vi "SensorInterface_Main.vi"(8 "error in (no error)":errorcluster) -> (0 "error out":errorcluster)   [LabVIEW 2013]
doc: "This is Top Level VI for Sensor Interface Module. You can communicate with this module using its API. Communication is made based on queue. This module has User Interface so I chase Producer Consumer architecture. In this architecture the User Interface loop is closed using User Event. User Event is sent by Processing (Consumer) loop."
uses:
  General/Controls/#TD_General_CommunicationQueueStates_Enum.ctl
  Private controls/#TD_SensorInterface_InnerData_Cluster.ctl
  Private controls/#TD_SensorInterface_ModuleStates_Enum.ctl
  Private controls/#TD_SensorInterface_ModuleData_Cluster.ctl
  General/Controls/#TD_General_FromWho_Enum.ctl
  General/Controls/#TD_General_UserEventStates_Enum.ctl
panel:
  in  "Funds Dispensed":bool
  in  "DepositReceived":bool
  # "[Covers: UI4] \n[Covers: UI4A] \n[Covers: UI4B]"
  # "[Covers: UI1]"
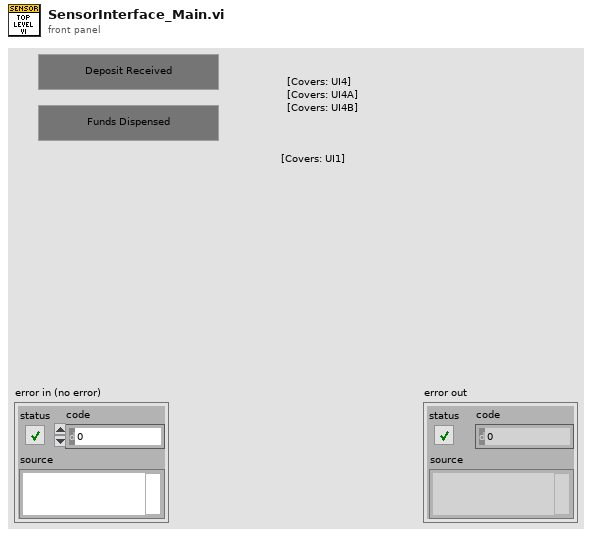
[diagram p1: front panel]
types:
  T1 = typedef "#TD_General_UserEventStates_Enum.ctl" = enum16{"ERROR_Default", "Create", "GetRef", "Generate", "Release"}
  T2 = typedef "#TD_General_CommunicationQueueStates_Enum.ctl" = enum16{"ERROR_Default", "Obtain", "GetRef", "Enqueue", "EnqueueAtOpp", "GetStatus", "Release"}
  T3 = typedef "#TD_General_FromWho_Enum.ctl" = enum16{"ERROR_Default", "UserConsole", "DisplayConsole", "SensorInterface", "Controller", "Database", "Timing", "ErrorHandling"}
  T4 = typedef "#TD_SensorInterface_ModuleStates_Enum.ctl" = enum16{"ERROR_Default", "Init", "Close", "ErrorHandling", "DepositReceived", "FundsDispensed"}
  T5 = typedef "#TD_SensorInterface_ModuleData_Cluster.ctl" = cluster{"Action":T4, "Data":variant}
  T6 = typedef "#TD_General_IntermoduleData_Cluster.ctl" = cluster{"Sender":T3, "ModuleData":variant}
  T7 = typedef "#TD_SensorInterface_InnerData_Cluster.ctl" = cluster{"Sth":bool}
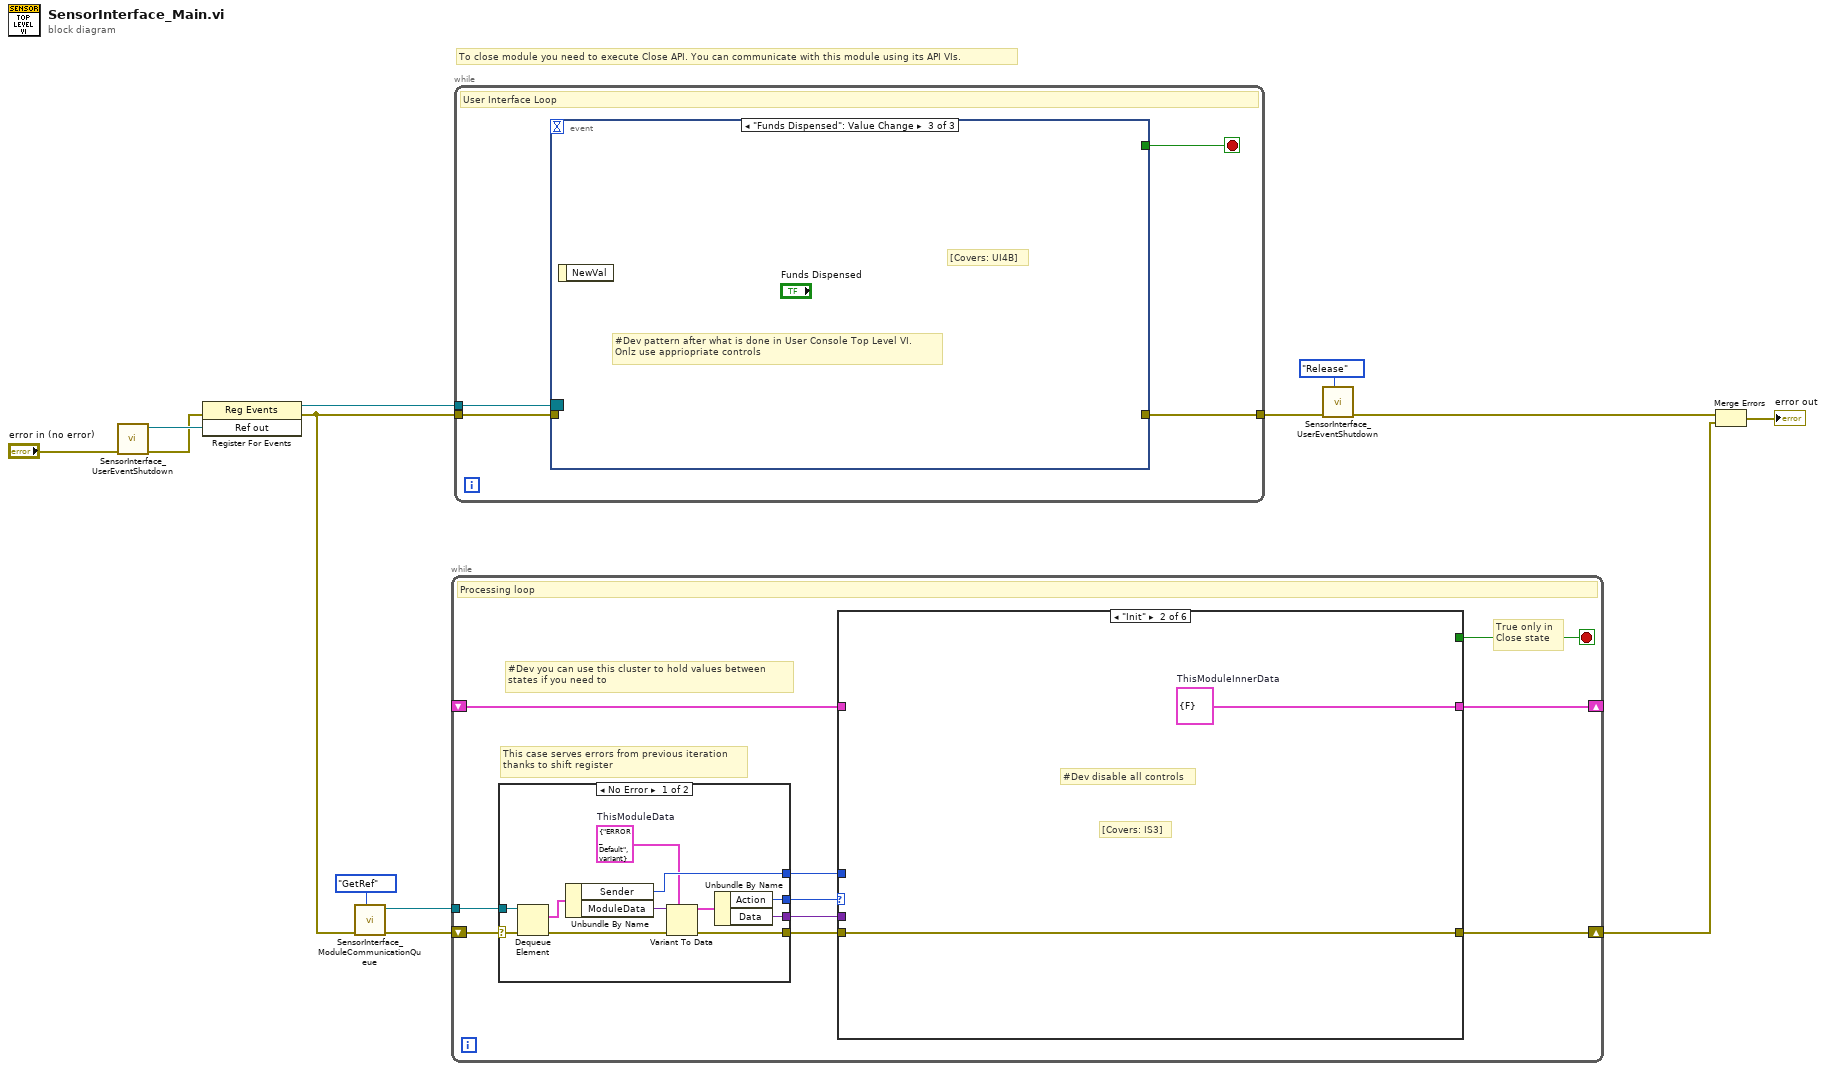
[diagram p0: block diagram]
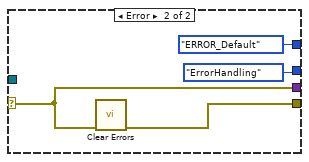
[diagram p2: hidden frame]
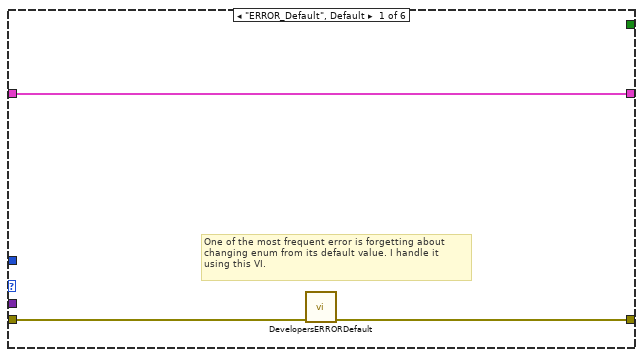
[diagram p3: hidden frame]
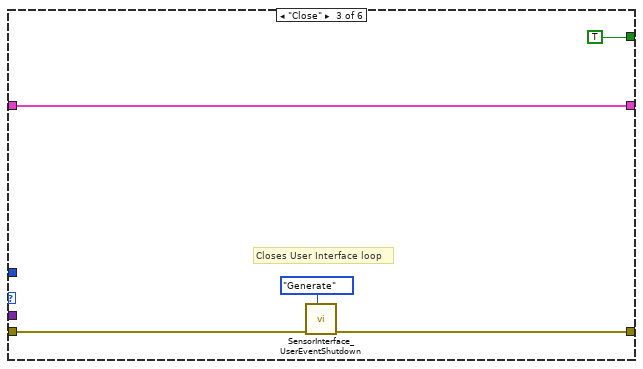
[diagram p4: hidden frame]
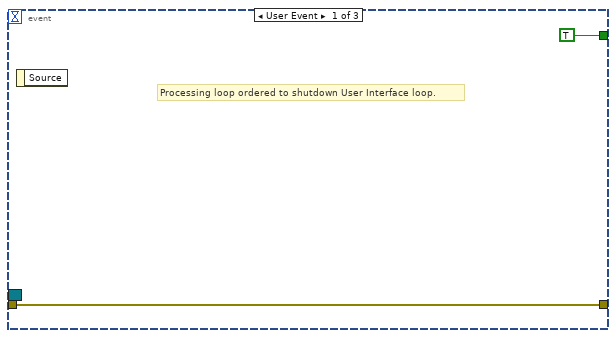
[diagram p8: hidden frame]
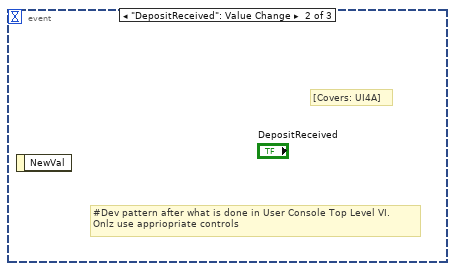
[diagram p9: hidden frame]
diagram:
  # "To close module you need to execute Close API. You can communicate with this module using its API VIs."
  n1 = call "SensorInterface_UserEventShutdown.vi"("error in (no error)"="error in (no error)") -> ("error out"=w12:errorcluster, "Ref out"=w13:refnum<user-event>)  [unwired: 9 in]
  n2 = register-events(error in=w12, w13) -> (reference out=w11:refnum<event-registration>, error out=w9:errorcluster)  [unwired: 1 in]
  n3 = call "SensorInterface_ModuleCommunicationQueue.vi"("Action"=#TD_General_CommunicationQueueStates_Enum."GetRef", "error in (no error)"=w9) -> ("error out"=w1:errorcluster, "Ref out"=w7:refnum<queue>)  [unwired: 7 in, 1 out]
  n4 = while {
    tunnel: w7 -> [w22]
    shift-right: [w15] -> w3
    shift-left: w1 -> [w23]
    shift-right: [w21] -> _
    shift-left: _ -> [w20]
    stop <- w14 stop-if-true
    # "True only in \nClose state"
    # "#Dev you can use this cluster to hold values between \nstates if you need to"
    # "This case serves errors from previous iteration \nthanks to shift register"
    # "Processing loop"
    n5 = case shown="No Error" w23 {
      selector: w23 -> [w34 w38]
      tunnel: w22 -> [w33 _]
      tunnel: [w29 #TD_General_FromWho_Enum."ERROR_Default" ("Sender")] -> w19
      tunnel: [w26 #TD_SensorInterface_ModuleStates_Enum."ErrorHandling" ("Action")] -> w18
      tunnel: [w25 w38] -> w17
      tunnel: [w24 w37] -> w16
      frame No Error {
        w28 = T5 {"Action"=enum."ERROR_Default", "Data"=variant}  # ThisModuleData
        n6 = Dequeue Element(queue=w33, error in (no error)=w34) -> (element=w32:T6, error out=w30:errorcluster)  [unwired: 1 in, 2 out]
        n7 = Unbundle By Name(w32) -> ("Sender"=w29:T3, "ModuleData"=w31:variant)
        n8 = Variant To Data(error in=w30, type=w28, Variant=w31) -> (data=w27:T5, error out=w24:errorcluster)
        n9 = Unbundle By Name(w27) -> ("Action"=w26:T4, "Data"=w25:variant)
      }
      frame Error {
        n10 = call <vilib>:"Clear Errors.vi"("error in (no error)"=w38) -> ("error out"=w37:errorcluster)  [unwired: 5 in, 1 out]
      }
    }
    n11 = case shown="\"Init\"" w18 {
      tunnel: [w41 w43 w47 w50 _ _] -> w21
      tunnel: w20 -> [w41 _ w47 w50 _ _]
      tunnel: w19 -> [_ _ _ _ _ _]
      tunnel: w17 -> [_ _ _ _ _ _]
      tunnel: w16 -> [w40 w42 w46 w49 _ _]
      tunnel: [w39 w42 w45 w49 _ _] -> w15
      tunnel: [_ _ TRUE _ _ _] -> w14
      frame "ERROR_Default", Default {
        # "One of the most frequent error is forgetting about \nchanging enum from its default value. I handle it \nusing this VI."
        n12 = call "DevelopersERRORDefault.vi"("error in (no error)"=w40) -> ("error out"=w39:errorcluster)  [unwired: 10 in]
      }
      frame "Init" {
        w43 = T7 {"Sth"=FALSE}  # ThisModuleInnerData
        # "[Covers: IS3]"
        # "#Dev disable all controls"
      }
      frame "Close" {
        # "Closes User Interface loop"
        n13 = call "SensorInterface_UserEventShutdown.vi"("Action"=#TD_General_UserEventStates_Enum."Generate", "error in (no error)"=w46) -> ("error out"=w45:errorcluster)  [unwired: 8 in, 1 out]
      }
      frame "ErrorHandling" {
        # "#Dev take some actions to handle the error \nand inform central Error Handling Module \nabout this error using Error Handling Module \nAPI"
      }
      frame "DepositReceived" {
        # "[Covers: UI4A]"
        # "#Dev using Controller's API send information about Deposit Received pressed \nto te controller"
      }
      frame "FundsDispensed" {
        # "[Covers: UI4B]"
        # "#Dev using Controller Module's API send infom to the Controller \nabout Funds Dispensed button Pressed"
      }
    }
  }
  n14 = while {
    tunnel: w11 -> [w54]
    tunnel: w9 -> [w52]
    tunnel: [w51] -> w6
    stop <- w53 stop-if-true
    # "User Interface Loop"
    n15 = event shown="[2] \"Funds Dispensed\": Value Change" {
      selector: w54 -> [_ _ _]
      dyn-events: _ -> [_ _ _]
      timeout: _ -> [_ _ _]
      tunnel: [TRUE _ _] -> w53
      tunnel: w52 -> [w55 _ _]
      tunnel: [w55 _ _] -> w51
      event User Event {
        # "Processing loop ordered to shutdown User Interface loop."
        n16 = event-data() -> ()  [unwired: 1 in, 1 out]
      }
      event "DepositReceived": Value Change {
        # "[Covers: UI4A]"
        # "#Dev pattern after what is done in User Console Top Level VI. \nOnlz use appriopriate controls"
        n17 = event-data() -> ()  [unwired: 1 in, 1 out]
      }
      event "Funds Dispensed": Value Change {
        # "[Covers: UI4B]"
        # "#Dev pattern after what is done in User Console Top Level VI. \nOnlz use appriopriate controls"
        n18 = event-data() -> ()  [unwired: 1 in, 1 out]
      }
    }
  }
  n19 = call "SensorInterface_UserEventShutdown.vi"("Action"=#TD_General_UserEventStates_Enum."Release", "error in (no error)"=w6) -> ("error out"=w4:errorcluster)  [unwired: 8 in, 1 out]
  n20 = Merge Errors(w4, w3) -> (→"error out":errorcluster)
